vi "encoder_test_3mode_v1.vi"() -> ()   [LabVIEW 2014]
uses:
  <vilib>/rvi/FXPMathLib/FxpSinAndCos/subVIs/nifxpmath_SinAndCos_SimConfig.ctl
  <vilib>/rvi/Emulation/niFpgaGetClockAttributes.vi
  <vilib>/rvi/Emulation/niFpgaSctlEmulationGetInTimedLoop.vi
  <vilib>/rvi/Emulation/niFpgaEmulationReportErrorSimple.vi
  <vilib>/rvi/eio/common/nirviEmuTemplateMethod_errors.vi
  <vilib>/rvi/Emulation/niFpgaProcessEmulError.vi
  <vilib>/rvi/Emulation/niFpgaCriticalErrorInLSC.vi
  <vilib>/rvi/FXPMathLib/FxpSinAndCos/simVIs/DllFxpSinAndCosTemp_sub.vi
  <vilib>/rvi/interface/RandomDataEmulation/nirviRandomDataMultiElementFPGAFIFO.vi
  <instcachedir>/0/nirviRandomDataMultiElementFPGAFIFO_AD0CFC12EF974623A9C2E4184BC062B2.lvgen/nirviRandomDataMultiElementFPGAFIFO_AD0CFC12EF974623A9C2E4184BC062B2_020.vi
  <vilib>/rvi/interface/RandomDataEmulation/niFpgaRandomDataHandleErrors.vi
  <vilib>/eio/EIONode/EIONode.xnode
  <vilib>/rvi/FXPMathLib/FxpMul/XNode/nifxpmath_Multiplier.xnode
  <vilib>/rvi/FXPMathLib/FxpSinAndCos/XNode/nifxpmath_SinAndCos.xnode
  <vilib>/rvi/Analysis/measure/butterworth/XNode/niFpgaButterworthFilter.xnode
  <vilib>/rvi/FXPMathLib/FxpSub/XNode/nifxpmath_Sub.xnode
  <vilib>/rvi/FXPMathLib/FxpAdd/XNode/nifxpmath_Add.xnode
  <vilib>/rvi/DataTransferAndStorage/Container/XNode/niFpgaContainer.xnode
  <vilib>/rvi/interface/RandomDataEmulation/nirviRandomDataFpgaMultiElementTemplate.vi
  <vilib>/rvi/FXPMathLib/sim/FxpSim.dll
panel:
  out "Dr_ramp":fxp<+/-,64,30>
  out "Dr_slope":fxp<+/-,33,17>
  in  "Dr_time":fxp<+/-,16,11>
  out "Dr_sin":fxp<+/-,28,11>
  out "Dr_sin_d":fxp<+/-,64,16>
  out "Dr_sin_dd":fxp<+/-,64,25>
  out "Sin omega":fxp<+/-,41,8>
  in  "Sin offset":fxp<+/-,27,10>
  in  "Sin magnitude":fxp<+/-,11,8>
  in  "Sin wave frequency (Hz)":fxp<+/-,21,5>
  out "Time now (s)":fxp<+,52,14>
  out "Dr":fxp<+/-,64,30>
  in  "Dr_end":fxp<+/-,16,11>
  in  "Command type":i16(ring) items=["Step", "Ramp", "Sine"]
  out "D_i":fxp<+/-,34,18>
  in  "D_tolorence":fxp<+/-,14,3>
  in  "Ki":fxp<+/-,20,6>
  out "D_error":fxp<+/-,24,11>
  in  "Direction":bool
  out "Fmr_PD":fxp<+/-,64,31>
  in  "Kd":fxp<+/-,20,8>
  in  "Kp":fxp<+/-,20,12>
  in  "scaled coefficients_D_dd":i32[](array[numeric])=[780119100, 146811362]
  out "D_dd":fxp<+/-,36,29>
  in  "Ini coe.":bool
  out "va":fxp<+/-,38,8>
  out "vb":fxp<+/-,38,8>
  in  "stop motor":bool
  out "vq_F":fxp<+/-,20,5> format="%.57g"
  out "vd_F":fxp<+/-,20,5>
  out "D_d (mm/s)":fxp<+/-,32,12>
  out "mt":u32
  out "omega (rad/s)":fxp<+/-,32,18>
  in  "mt0":u32
  out "D(mm)":fxp<+/-,22,7>
  out "rad(NrTheta)":fxp<+/-,33,18>
  out "Encoder Position":i32
  in  "Encoder Reset":bool
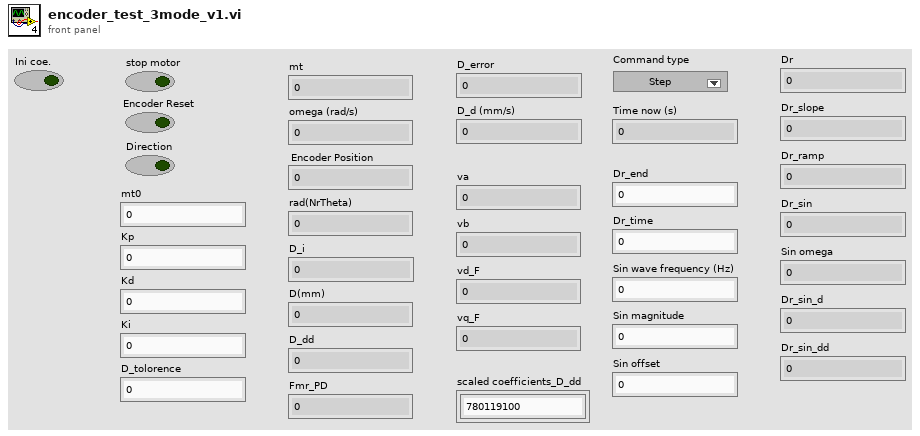
[diagram p1: front panel]
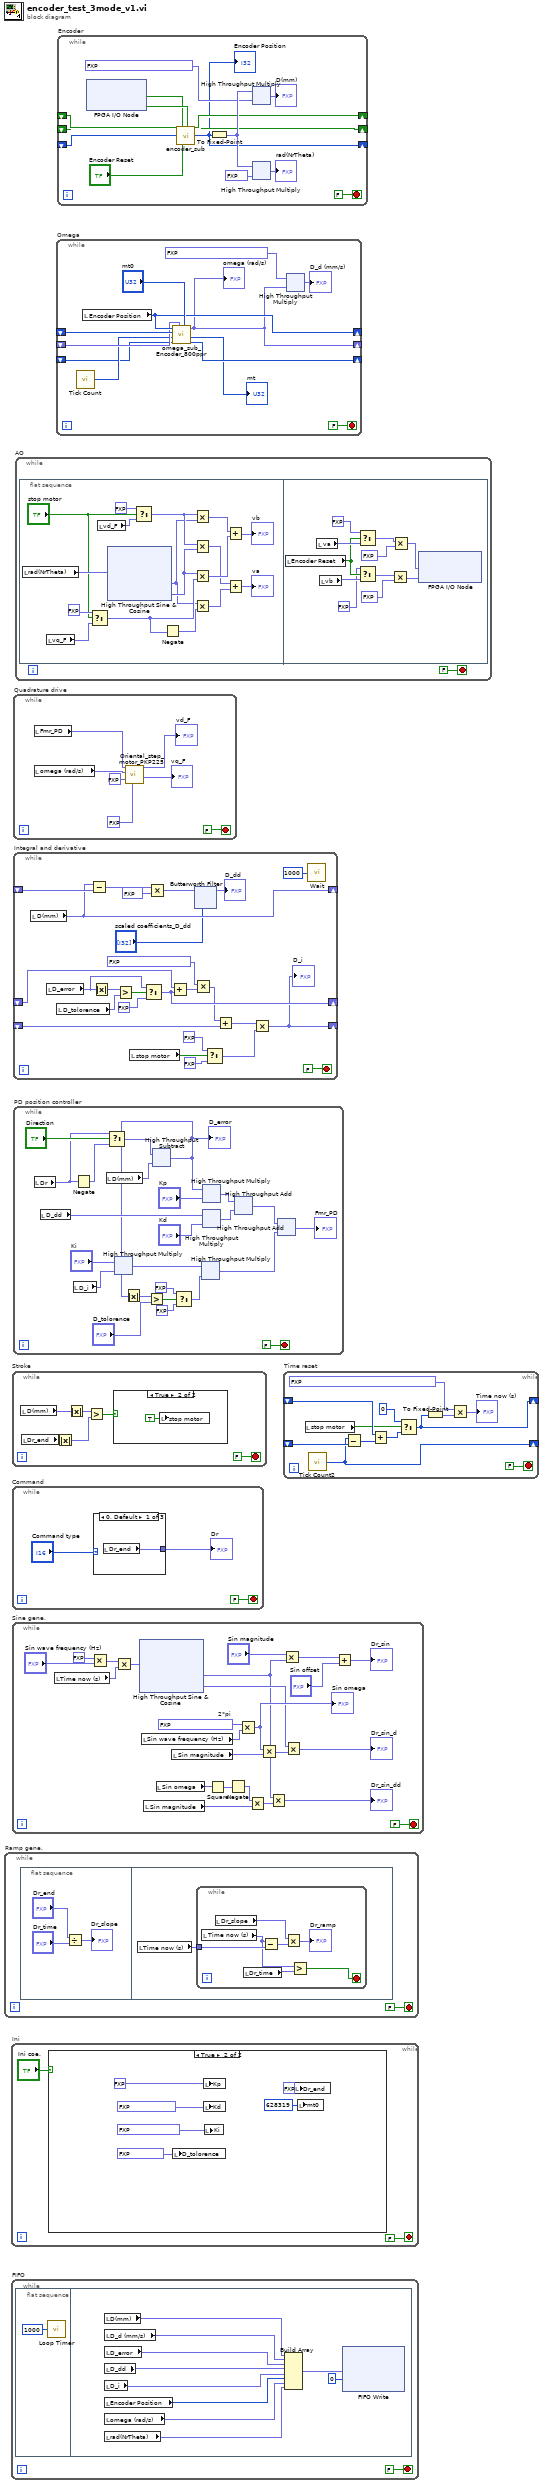
[diagram p0: block diagram]
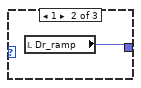
[diagram p2: hidden frame]
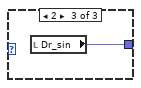
[diagram p3: hidden frame]
diagram:
  n1 = while "Ramp gene." {
    stop <- FALSE stop-if-true
    n2 = flat-sequence {
      frame #0 {
        n3 = Divide(x="Dr_end", y="Dr_time") -> (x/y=→"Dr_slope":fxp<+/-,33,17>)
      }
      frame #1 {
        n4 = local read "Time now (s)"() -> (w5:fxp<+,52,14>)
        n5 = while {
          tunnel: w5 -> [w12]
          stop <- w6 stop-if-true
          n6 = local read "Time now (s)"() -> (w7:fxp<+,52,14>)
          n7 = local read "Dr_slope"() -> (w10:fxp<+/-,33,17>)
          n8 = local read "Dr_time"() -> (w8:fxp<+/-,16,11>)
          n9 = Subtract(x=w7, y=w12) -> (x-y=w11:fxp<+/-,53,15>)
          n10 = Multiply(x=w10, y=w11) -> (x*y=→"Dr_ramp":fxp<+/-,64,30>)
          n11 = Greater?(x=w7, y=w8) -> (0:w6:bool)
        }
      }
    }
  }
  n12 = while "Ini" {
    stop <- FALSE stop-if-true
    n13 = case shown="True" "Ini coe." {
      frame False {
      }
      frame True {
        n14 = local write "D_tolorence"(fxp<+/-,14,3> 0.009765625 ("D_tolorence")) -> ()
        n15 = local write "Kp"(fxp<+/-,20,12> 2.0 ("Kp")) -> ()
        n16 = local write "Kd"(fxp<+/-,20,8> 1.800048828125 ("Kd")) -> ()
        n17 = local write "Ki"(fxp<+/-,20,6> 0.0999755859375 ("D_i")) -> ()
        n18 = local write "Dr_end"(fxp<+/-,11,7> 20.0 ("Fmr")) -> ()
        n19 = local write "mt0"(u32 628319 ("mt0")) -> ()
      }
    }
  }
  n20 = while "FIFO" {
    stop <- FALSE stop-if-true
    n21 = flat-sequence {
      frame #0 {
        n22 = call "Loop Timer"("Count(uSec)"=u32 1000) -> ()  [unwired: 1 out]
      }
      frame #1 {
        n23 = local read "D(mm)"() -> (w30:fxp<+/-,22,7>)
        n24 = local read "D_d (mm/s)"() -> (w29:fxp<+/-,32,12>)
        n25 = local read "D_error"() -> (w28:fxp<+/-,24,11>)
        n26 = local read "D_dd"() -> (w27:fxp<+/-,36,29>)
        n27 = local read "D_i"() -> (w26:fxp<+/-,34,18>)
        n28 = local read "Encoder Position"() -> (w25:i32)
        n29 = local read "omega (rad/s)"() -> (w24:fxp<+/-,32,18>)
        n30 = local read "rad(NrTheta)"() -> (w23:fxp<+/-,33,18>)
        n31 = Build Array(w30, w29, w28, w27, w26, w25, w24, w23) -> (w31:fxp<+/-,52,32>[])
        n32 = xnode ("FIFO Write")("Element"=w31, "Timeout"=0) -> ()  [unwired: 1 in, 2 out]
      }
    }
  }
  n33 = while "Stroke" {
    stop <- FALSE stop-if-true
    n34 = local read "D(mm)"() -> (w38:fxp<+/-,22,7>)
    n35 = local read "Dr_end"() -> (w34:fxp<+/-,16,11>)
    n36 = Absolute Value(x=w34) -> (abs(x)=w33:fxp<+,16,11>)
    n37 = Absolute Value(x=w38) -> (abs(x)=w37:fxp<+,22,7>)
    n38 = Greater?(x=w37, y=w33) -> (0:w36:bool)
    n39 = case shown="True" w36 {
      frame False {
      }
      frame True {
        n40 = local write "stop motor"(TRUE ("stop motor")) -> ()
      }
    }
  }
  n41 = while "Command" {
    stop <- FALSE stop-if-true
    n42 = case shown="0, Default" "Command type" {
      tunnel: [w43 w44 w45] -> w41
      frame 0, Default {
        n43 = local read "Dr_end"() -> (w43:fxp<+/-,16,11>)
      }
      frame 1 {
        n44 = local read "Dr_ramp"() -> (w44:fxp<+/-,64,30>)
      }
      frame 2 {
        n45 = local read "Dr_sin"() -> (w45:fxp<+/-,28,11>)
      }
    }
    "Dr" <- w41
  }
  n46 = while "Sine gene." {
    stop <- FALSE stop-if-true
    w63 = fxp<+,20,3> 6.2831878662109375  # 2*pi
    n47 = local read "Time now (s)"() -> (w66:fxp<+,52,14>)
    n48 = Multiply(x=fxp<+,1,2> 2.0, y="Sin wave frequency (Hz)") -> (x*y=w67:fxp<+/-,21,6>)
    n49 = Multiply(x=w67, y=w66) -> (x*y=w47:fxp<+/-,64,20>)
    n50 = xnode "High Throughput Sine & Cosine"("x (pi)"=w47) -> ("sin(x)"=w51:fxp<+/-,16,2>, "cos(x)"=w58:fxp<+/-,16,2>)
    n51 = local read "Sin wave frequency (Hz)"() -> (w62:fxp<+/-,21,5>)
    n52 = local read "Sin magnitude"() -> (w53:fxp<+/-,11,8>)
    n53 = local read "Sin omega"() -> (w54:fxp<+/-,41,8>)
    n54 = local read "Sin magnitude"() -> (w57:fxp<+/-,11,8>)
    n55 = Square(x=w54) -> (x^2=w55:fxp<+,64,14>)
    n56 = Negate(x=w55) -> (-x=w52:fxp<+/-,64,15>)
    n57 = Multiply(x=w63, y=w62) -> (x*y=w59:fxp<+/-,41,8>)
    "Sin omega" <- w59
    n58 = Multiply(x=w52, y=w53) -> (x*y=w56:fxp<+/-,64,23>)
    n59 = Multiply(x=w59, y=w57) -> (x*y=w64:fxp<+/-,51,15>)
    n60 = Multiply(x=w51, y=w56) -> (x*y=→"Dr_sin_dd":fxp<+/-,64,25>)
    n61 = Multiply(x="Sin magnitude", y=w51) -> (x*y=w65:fxp<+/-,27,10>)
    n62 = Multiply(x=w58, y=w64) -> (x*y=→"Dr_sin_d":fxp<+/-,64,16>)
    n63 = Add(x=w65, y="Sin offset") -> (x+y=→"Dr_sin":fxp<+/-,28,11>)
  }
  n64 = while "Quadrature drive" {
    stop <- FALSE stop-if-true
    n65 = local read "Fmr_PD"() -> (w100:fxp<+/-,64,31>)
    n66 = local read "omega (rad/s)"() -> (w102:fxp<+/-,32,18>)
    n67 = call "Oriental_step_motor_PKP225.vi"("F_Threshold"=fxp<+,12,12> 10.0, "dFmr"=fxp<+/-,25,15> 0.0, "omega"=w102, "Fmr"=w100) -> ("vq_F"=→"vq_F":fxp<+/-,20,5>, "vd_F"=→"vd_F":fxp<+/-,20,5>)  [unwired: 6 in]
  }
  n68 = while "Integral and derivative" {
    shift-right: [w127] -> _
    shift-left: _ -> [w131]
    shift-right: [w117] -> _
    shift-left: _ -> [w118]
    shift-right: [w107] -> _
    shift-left: _ -> [w111]
    stop <- FALSE stop-if-true
    n69 = local read "D(mm)"() -> (w127:fxp<+/-,22,7>)
    n70 = local read "D_error"() -> (w119:fxp<+/-,24,11>)
    n71 = local read "D_tolorence"() -> (w122:fxp<+/-,14,3>)
    n72 = Subtract(x=w127, y=w131) -> (x-y=w130:fxp<+/-,23,8>)
    n73 = Absolute Value(x=w119) -> (abs(x)=w123:fxp<+,24,11>)
    n74 = Greater?(x=w123, y=w122) -> (0:w121:bool)
    n75 = local read "stop motor"() -> (w114:bool)
    n76 = Select(t=w119, s=w121, f=fxp<+,24,11> 0.0) -> (s? t:f=w117:fxp<+/-,25,12>)
    n77 = Multiply(x=w130, y=fxp<+/-,33,13> 1000.0) -> (x*y=w128:fxp<+/-,55,20>)
    n78 = Add(x=w118, y=w117) -> (x+y=w116:fxp<+/-,26,13>)
    n79 = Multiply(x=fxp<+/-,30,12> 0.000499725341796875, y=w116) -> (x*y=w110:fxp<+/-,55,24>)
    n80 = xnode "Butterworth Filter"("input data"=w128, "scaled coefficients"="scaled coefficients_D_dd") -> ("output data"=→"D_dd":fxp<+/-,36,24>)  [unwired: 1 in]
    n81 = Select(t=fxp<+,1,1> 0.0, s=w114, f=fxp<+,1,1> 1.0) -> (s? t:f=w108:fxp<+,1,1>)
    n82 = Add(x=w110, y=w111) -> (x+y=w109:fxp<+/-,32,16>)
    n83 = Multiply(x=w109, y=w108) -> (x*y=w107:fxp<+/-,32,16>)
    "D_i" <- w107
    n84 = call "Wait"("Count(uSec)"=u32 1000) -> ()  [unwired: 1 out]
  }
  n85 = while "PD position controller" {
    stop <- FALSE stop-if-true
    n86 = local read "Dr"() -> (w141:fxp<+/-,64,30>)
    n87 = local read "D_dd"() -> (w160:fxp<+/-,36,29>)
    n88 = local read "D_i"() -> (w152:fxp<+/-,34,18>)
    n89 = Negate(x=w141) -> (-x=w156:fxp<+/-,64,31>)
    n90 = local read "D(mm)"() -> (w164:fxp<+/-,22,7>)
    n91 = Select(t=w141, s="Direction", f=w156) -> (s? t:f=w155:fxp<+/-,64,31>)
    n92 = xnode ("High Throughput Multiply")("x"="Ki", "y"=w152) -> ("x*y"=w146:fxp<+/-,54,24>)
    n93 = xnode "High Throughput Subtract"("x"=w155, "y"=w164) -> ("x-y"=w150:fxp<+/-,64,32>)
    "D_error" <- w150
    n94 = Absolute Value(x=w150) -> (abs(x)=w151:fxp<+,64,32>)
    n95 = Greater?(x=w151, y="D_tolorence") -> (0:w149:bool)
    n96 = Select(t=fxp<+,10,2> 1.0, s=w149, f=fxp<+,10,2> 0.0) -> (s? t:f=w145:fxp<+,10,2>)
    n97 = xnode ("High Throughput Multiply")("x"=w146, "y"=w145) -> ("x*y"=w142:fxp<+/-,64,26>)
    n98 = xnode ("High Throughput Multiply")("x"=w150, "y"="Kp") -> ("x*y"=w162:fxp<+/-,64,44>)
    n99 = xnode ("High Throughput Multiply")("x"=w160, "y"="Kd") -> ("x*y"=w161:fxp<+/-,56,37>)
    n100 = xnode ("High Throughput Add")("x"=w162, "y"=w161) -> ("x+y"=w143:fxp<+/-,64,45>)
    n101 = xnode ("High Throughput Add")("x"=w143, "y"=w142) -> ("x+y"=→"Fmr_PD":fxp<+/-,64,46>)
  }
  n102 = while "AO" {
    stop <- FALSE stop-if-true
    n103 = flat-sequence {
      frame #0 {
        n104 = local read "rad(NrTheta)"() -> (w181:fxp<+/-,33,18>)
        n105 = local read "vq_F"() -> (w179:fxp<+/-,20,5>)
        n106 = Select(t=fxp<+,20,5> 0.0, s="stop motor", f=w179) -> (s? t:f=w176:fxp<+/-,21,6>)
        n107 = local read "vd_F"() -> (w180:fxp<+/-,20,5>)
        n108 = xnode "High Throughput Sine & Cosine"("x (pi)"=w181) -> ("sin(x)"=w172:fxp<+/-,17,2>, "cos(x)"=w174:fxp<+/-,17,2>)
        n109 = Select(t=fxp<+,20,5> 0.0, s="stop motor", f=w180) -> (s? t:f=w173:fxp<+/-,21,6>)
        n110 = Negate(x=w176) -> (-x=w175:fxp<+/-,21,6>)
        n111 = Multiply(x=w173, y=w172) -> (x*y=w171:fxp<+/-,37,7>)
        n112 = Multiply(x=w173, y=w174) -> (x*y=w169:fxp<+/-,37,7>)
        n113 = Multiply(x=w174, y=w176) -> (x*y=w170:fxp<+/-,37,7>)
        n114 = Multiply(x=w172, y=w175) -> (x*y=w168:fxp<+/-,37,7>)
        n115 = Add(x=w171, y=w170) -> (x+y=→"vb":fxp<+/-,38,8>)
        n116 = Add(x=w169, y=w168) -> (x+y=→"va":fxp<+/-,38,8>)
      }
      frame #1 {
        n117 = local read "Encoder Reset"() -> (w215:bool)
        n118 = local read "va"() -> (w217:fxp<+/-,38,8>)
        n119 = local read "vb"() -> (w216:fxp<+/-,38,8>)
        n120 = Select(t=fxp<+/-,20,5> 5.0 ("y"), s=w215, f=w217) -> (s? t:f=w218:fxp<+/-,38,8>)
        n121 = Select(t=fxp<+/-,20,5> 0.0 ("y"), s=w215, f=w216) -> (s? t:f=w219:fxp<+/-,38,8>)
        n122 = Multiply(x=w219, y=fxp<+/-,20,5> -0.5) -> (x*y=w223:fxp<+/-,57,12>)
        n123 = Multiply(x=w218, y=fxp<+/-,20,5> -0.5) -> (x*y=w222:fxp<+/-,57,12>)
        n124 = xnode "FPGA I/O Node"("Mod8/AO0"=w222, "Mod8/AO1"=w223) -> ()  [unwired: 2 in, 2 out]
      }
    }
  }
  n125 = while "Omega" {
    shift-right: [w233] -> _
    shift-left: _ -> [w234]
    shift-right: [w226] -> _
    shift-left: _ -> [w232]
    shift-right: [w229] -> _
    shift-left: _ -> [w230]
    stop <- FALSE stop-if-true
    n126 = call "Tick Count"() -> ("Tick Count(Ticks)"=w231:u32)
    n127 = local read "Encoder Position"() -> (w233:i32)
    n128 = call "omega_sub_Encoder_800ppr.vi"("mt0"="mt0", "omega_pre"=w232, "ticks_m_pre"=w230, "ticks"=w231, "count_pre"=w234, "count"=w233) -> ("ticks_m"=w229:u32, "mt"=→"mt":u32, "omega"=w226:fxp<+/-,20,9>)  [unwired: 3 in]
    "omega (rad/s)" <- w226
    n129 = xnode ("High Throughput Multiply")("x"=fxp<+/-,26,1> 0.3183099031448364, "y"=w226) -> ("x*y"=→"D_d (mm/s)":fxp<+/-,46,10>)
  }
  n130 = while "Encoder" {
    shift-right: [w242] -> _
    shift-left: _ -> [w244]
    shift-right: [w241] -> _
    shift-left: _ -> [w243]
    shift-right: [w239] -> _
    shift-left: _ -> [w240]
    stop <- FALSE stop-if-true
    n131 = xnode "FPGA I/O Node"() -> ("Mod4/DI3"=w249:bool, "Mod4/DI4"=w250:bool)  [unwired: 2 in, 2 out]
    n132 = call "encoder_sub.vi"("A_pre"=w244, "B_pre"=w243, "Encoder Position_pre"=w240, "A input"=w249, "Encoder Position Reset"="Encoder Reset", "B input"=w250) -> ("A"=w242:bool, "B"=w241:bool, "Encoder Position (Counts)"=w239:i32)  [unwired: 19 in]
    "Encoder Position" <- w239
    n133 = To Fixed-Point(number=w239) -> (fixed-point=w247:fxp<+/-,32,32>)  [unwired: 1 in]
    n134 = xnode ("High Throughput Multiply")("x"=w247, "y"=fxp<+/-,24,0> 0.002499997615814209) -> ("x*y"=→"D(mm)":fxp<+/-,56,32>)
    n135 = xnode ("High Throughput Multiply")("x"=w247, "y"=fxp<+/-,24,0> 0.125) -> ("x*y"=→"rad(NrTheta)":fxp<+/-,56,32>)
  }
  n136 = while "Time reset" {
    shift-right: [w254] -> _
    shift-left: _ -> [w261]
    shift-right: [w256] -> _
    shift-left: _ -> [w257]
    stop <- FALSE stop-if-true
    n137 = local read "stop motor"() -> (w259:bool)
    n138 = call "Tick Count2"() -> ("Tick Count(uSec)"=w256:u32)
    n139 = Subtract(x=w256, y=w257) -> (x-y=w262:u32)
    n140 = Add(x=w261, y=w262) -> (x+y=w260:u32)
    n141 = Select(t=u32 0, s=w259, f=w260) -> (s? t:f=w254:u32)
    n142 = To Fixed-Point(number=w254) -> (fixed-point=w253:fxp<+,32,32>)  [unwired: 1 in]
    n143 = Multiply(x=fxp<+,20,-18> 1.0000003385357559e-06, y=w253) -> (x*y=→"Time now (s)":fxp<+,52,14>)
  }
